vi "take_data (SubVI).vi"(8 "instrum in":T1, 11 "channel settings":T3={"samples per channel"=1000, "sampling rate"=1000.0, "data task"="", "drive channel"="", "Clock src"="", "synth trigger"=""} {"sampling rate" format="%0.2f"}) -> (0 "instrum out":T1, 2 "data tasks":T2, 3 "Actual Sample Rate":dbl=10000.0 format="%0.2f")   [LabVIEW 2014]
uses:
  <vilib>/DAQmx/create/channels.llb/DAQmx Create Channel (AO-Voltage-Basic).vi
  <vilib>/DAQmx/configure/timing.llb/DAQmx Timing (Sample Clock).vi
  <vilib>/DAQmx/create/channels.llb/DAQmx Create Channel (AI-Voltage-Basic).vi
  <vilib>/DAQmx/configure/trigger.llb/DAQmx Start Trigger (Digital Edge).vi
  <vilib>/DAQmx/write.llb/DAQmx Write (Analog 1D DBL 1Chan NSamp).vi
  <resource>/objmgr/daqmx.rc
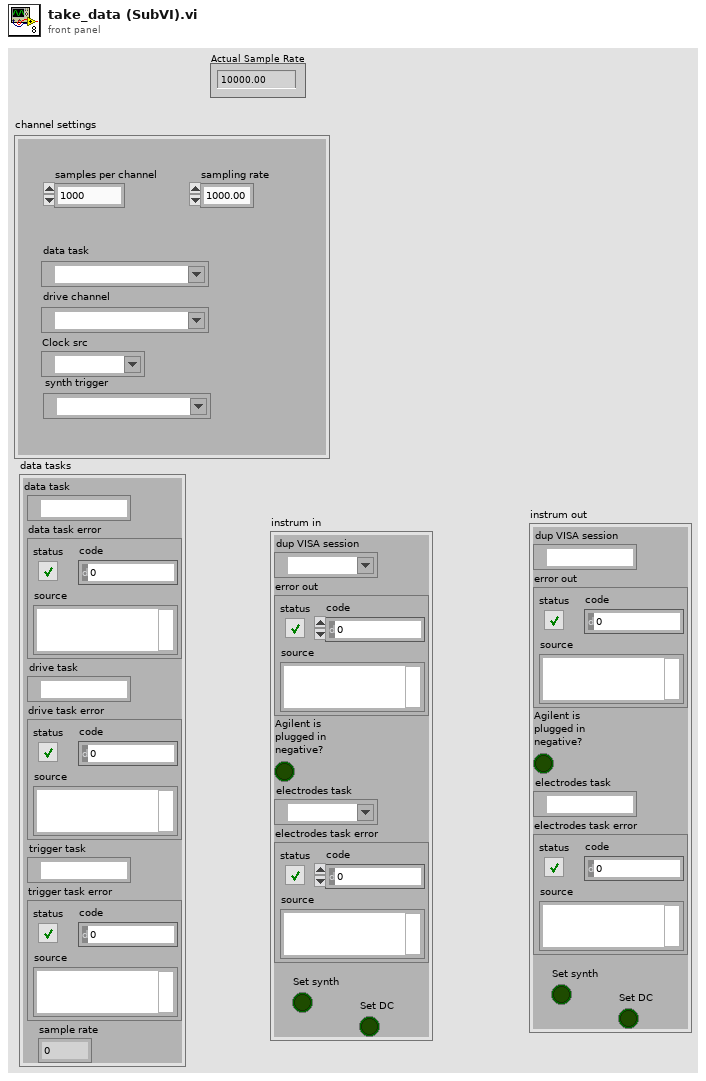
[diagram p1: front panel]
types:
  T1 = cluster{"dup VISA session":refnum<visa-resource-name>, "error out":errorcluster, "Agilent is \nplugged in \nnegative?":bool, "electrodes task":refnum<k21>, "electrodes task error":errorcluster, "Set synth":bool, "Set DC":bool}
  T2 = cluster{"data task":refnum<k21>, "data task error":errorcluster, "drive task":refnum<k21>, "drive task error":errorcluster, "trigger task":refnum<k21>, "trigger task error":errorcluster, "sample rate":dbl}
  T3 = cluster{"samples per channel":i32, "sampling rate":dbl, "data task":tag, "drive channel":tag, "Clock src":tag, "synth trigger":tag}
  T4 = cluster{"task out":refnum<k21>, "error out":errorcluster, "task out":refnum<k21>, "error out":errorcluster, "task out":refnum<k21>, "error out":errorcluster, "SampClk.Rate":dbl}
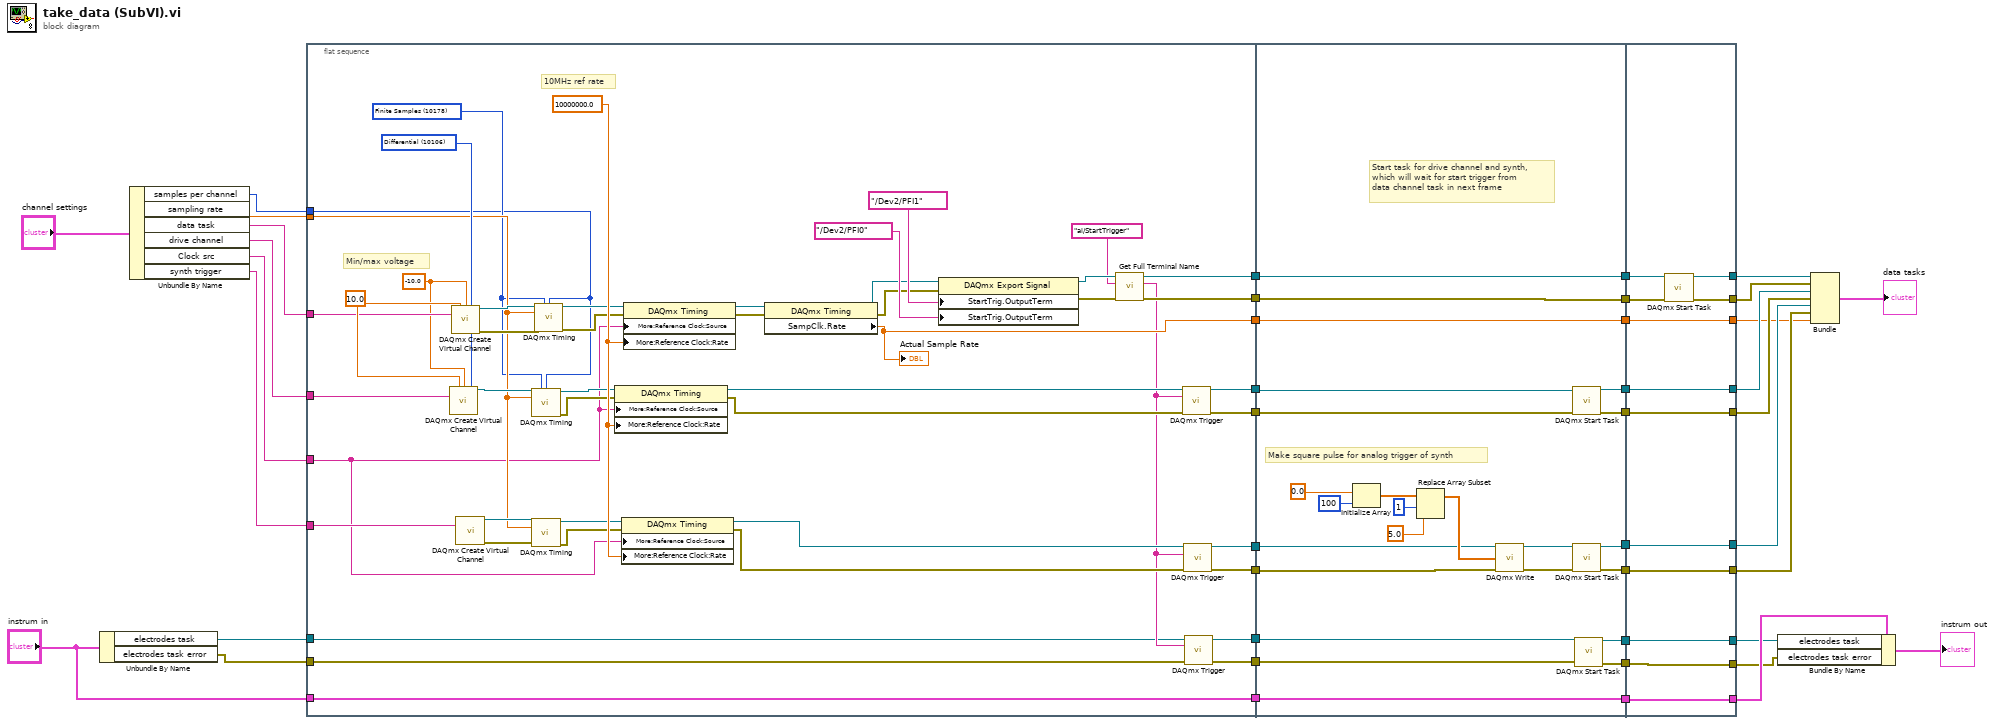
[diagram p0: block diagram]
diagram:
  n1 = Unbundle By Name("instrum in") -> ("electrodes task"=w13:refnum<k21>, "electrodes task error"=w12:errorcluster)
  n2 = Unbundle By Name("channel settings") -> ("samples per channel"=w36:i32, "sampling rate"=w38:dbl, "data task"=w41:tag, "drive channel"=w40:tag, "Clock src"=w37:tag, "synth trigger"=w39:tag)
  n3 = flat-sequence {
    tunnel: w41 -> [w63]
    tunnel: w40 -> [w62]
    tunnel: w39 -> [w61]
    tunnel: w38 -> [w59]
    tunnel: w37 -> [w57]
    tunnel: w36 -> [w56]
    tunnel: [w55] -> w35
    tunnel: [w54] -> w34
    tunnel: [w53] -> w33
    tunnel: [w52] -> w32
    tunnel: [w51] -> w31
    tunnel: [w50] -> w30
    tunnel: [w49] -> w17
    tunnel: w13 -> [w43]
    tunnel: w12 -> [w47]
    tunnel: [w46] -> w11
    tunnel: [w45] -> w10
    tunnel: "instrum in" -> [w44]
    tunnel: [w44] -> w7
    tunnel: w35 -> [w106]
    tunnel: w34 -> [w105]
    tunnel: w33 -> [w104]
    tunnel: w32 -> [w103]
    tunnel: w31 -> [w100]
    tunnel: w30 -> [w99]
    tunnel: [w106] -> w29
    tunnel: [w105] -> w28
    tunnel: [w102] -> w27
    tunnel: [w101] -> w26
    tunnel: [w98] -> w25
    tunnel: [w97] -> w24
    tunnel: w17 -> [w96]
    tunnel: [w96] -> w15
    tunnel: w11 -> [w95]
    tunnel: w10 -> [w94]
    tunnel: [w93] -> w8
    tunnel: w7 -> [w93]
    tunnel: [w92] -> w3
    tunnel: [w91] -> w2
    tunnel: w29 -> [w126]
    tunnel: w28 -> [w125]
    tunnel: w27 -> [w124]
    tunnel: w26 -> [w123]
    tunnel: [w124] -> w18
    tunnel: [w123] -> w19
    tunnel: [w122] -> w23
    tunnel: [w121] -> w22
    tunnel: w25 -> [w119]
    tunnel: w24 -> [w120]
    tunnel: [w120] -> w21
    tunnel: [w119] -> w20
    tunnel: [w118] -> w16
    tunnel: w15 -> [w118]
    tunnel: w8 -> [w117]
    tunnel: [w117] -> w6
    tunnel: [w116] -> w4
    tunnel: w3 -> [w116]
    tunnel: w2 -> [w115]
    tunnel: [w115] -> _
    tunnel: [w115] -> w1
    frame #0 {
      w60 = -10.0 ("minimum value")
      w64 = 10.0 ("maximum value")
      w65 = 10106 items=["default"=-1, "RSE"=10083, "NRSE"=10078, "Differential"=10106, "Pseudodifferential"=12529] ("input terminal configuration")
      w58 = 10178 items=["Finite Samples"=10178, "Continuous Samples"=10123, "Hardware Timed Single Point"=12522] ("sample mode")
      w88 = 10000000.0 ("RefClk.Rate")
      # "10MHz ref rate"
      # "Min/max voltage"
      n4 = call-poly <vilib>:"DAQmx Create Virtual Channel.vi"("maximum value"=w64, "minimum value"=w60, "input terminal configuration"=w65, "physical channels"=w62) -> ("task out"=w68:refnum<k21>)  [unwired: 10 in, 1 out]
      n5 = call-poly <vilib>:"DAQmx Create Virtual Channel.vi"("maximum value"=w64, "minimum value"=w60, "input terminal configuration"=w65, "physical channels"=w63) -> ("task out"=w66:refnum<k21>, "error out"=w67:errorcluster)  [unwired: 10 in]
      n6 = call-poly <vilib>:"DAQmx Create Virtual Channel.vi"("physical channels"=w61) -> ("task out"=w84:refnum<k21>, "error out"=w86:errorcluster)  [unwired: 13 in]
      n7 = call-poly <vilib>:"DAQmx Timing.vi"("task/channels in"=w68, "sample mode"=w58, "samples per channel"=w56, "rate"=w59) -> ("task out"=w71:refnum<k21>, "error out"=w72:errorcluster)  [unwired: 10 in]
      n8 = call-poly <vilib>:"DAQmx Timing.vi"("task/channels in"=w84, "rate"=w59, "error in"=w86) -> ("task out"=w85:refnum<k21>, "error out"=w87:errorcluster)  [unwired: 11 in]
      n9 = call-poly <vilib>:"DAQmx Timing.vi"("task/channels in"=w66, "sample mode"=w58, "samples per channel"=w56, "rate"=w59, "error in"=w67) -> ("task out"=w69:refnum<k21>, "error out"=w70:errorcluster)  [unwired: 9 in]
      n10 = property class="DAQmx Timing"(reference=w71, error in=w72, "More:Reference Clock:Source"=w57, "More:Reference Clock:Rate"=w88) -> (reference out=w76:refnum<k21>, error out=w77:errorcluster)
      n11 = property class="DAQmx Timing"(reference=w85, error in=w87, "More:Reference Clock:Source"=w57, "More:Reference Clock:Rate"=w88) -> (reference out=w90:refnum<k21>, error out=w89:errorcluster)
      n12 = property class="DAQmx Timing"(reference=w69, error in=w70, "More:Reference Clock:Source"=w57, "More:Reference Clock:Rate"=w88) -> (reference out=w73:refnum<k21>, error out=w74:errorcluster)
      n13 = property class="DAQmx Timing"(reference=w73, error in=w74) -> (reference out=w78:refnum<k21>, error out=w80:errorcluster, "SampClk.Rate"=w49:dbl)
      "Actual Sample Rate" <- w49
      n14 = property class="DAQmx Export Signal"(reference=w78, error in=w80, "StartTrig.OutputTerm"=tag "/Dev2/PFI1", "StartTrig.OutputTerm"=tag "/Dev2/PFI0" ("10MHzRefClk.OutputTerm")) -> (reference out=w79:refnum<k21>, error out=w81:errorcluster)
      n15 = call "Get Full Terminal Name.vi"("error in (no error)"=w81, "Local Terminal Name"="ai/StartTrigger", "task/channels in"=w79) -> ("error out"=w54:errorcluster, "Terminal Name with Device Prefix"=w48:tag, "task out"=w55:refnum<k21>)  [unwired: 6 in]
      n16 = call-poly <vilib>:"DAQmx Trigger.vi"("task/channels in"=w76, "source"=w48, "error in"=w77) -> ("task out"=w53:refnum<k21>, "error out"=w52:errorcluster)  [unwired: 11 in]
      n17 = call-poly <vilib>:"DAQmx Trigger.vi"("task/channels in"=w90, "source"=w48, "error in"=w89) -> ("task out"=w51:refnum<k21>, "error out"=w50:errorcluster)  [unwired: 11 in]
      n18 = call-poly <vilib>:"DAQmx Trigger.vi"("task/channels in"=w43, "source"=w48, "error in"=w47) -> ("task out"=w46:refnum<k21>, "error out"=w45:errorcluster)  [unwired: 11 in]
    }
    frame #1 {
      # "Start task for drive channel and synth,\nwhich will wait for start trigger from \ndata channel task in next frame"
      # "Make square pulse for analog trigger of synth"
      n19 = Initialize Array(0.0 ("element"), 100 ("dimension size")) -> (w109:dbl[])
      n20 = Replace Array Subset(array=w109, new element=5.0 ("new element/subarray"), index=1) -> (w112:dbl[])
      n21 = call-poly <vilib>:"DAQmx Write.vi"("task/channels in"=w100, "data"=w112, "error in"=w99) -> ("task out"=w111:refnum<k21>, "error out"=w110:errorcluster)  [unwired: 10 in, 1 out]
      n22 = call <vilib>:"DAQmx Start Task.vi"("task/channels in"=w104, "error in"=w103) -> ("task out"=w102:refnum<k21>, "error out"=w101:errorcluster)  [unwired: 12 in]
      n23 = call <vilib>:"DAQmx Start Task.vi"("task/channels in"=w111, "error in"=w110) -> ("task out"=w98:refnum<k21>, "error out"=w97:errorcluster)  [unwired: 12 in]
      n24 = call <vilib>:"DAQmx Start Task.vi"("task/channels in"=w95, "error in"=w94) -> ("task out"=w92:refnum<k21>, "error out"=w91:errorcluster)  [unwired: 12 in]
    }
    frame #2 {
      n25 = call <vilib>:"DAQmx Start Task.vi"("task/channels in"=w126, "error in"=w125) -> ("task out"=w122:refnum<k21>, "error out"=w121:errorcluster)  [unwired: 12 in]
    }
  }
  n26 = Bundle By Name(cluster=w6, "electrodes task"=w4, "electrodes task error"=w1) -> (→"instrum out":T1)
  n27 = Bundle("task out"=w23, "error out"=w22, "task out"=w18, "error out"=w19, "task out"=w20, "error out"=w21, "SampClk.Rate"=w16) -> (→"data tasks":T4)  [unwired: 1 in]
